vi "Filter And Analyze.vi"(9 "X Resolution":i32, 10 "Y Resolution":i32, 11 "Refnum in":T1) -> (0 "Number of Particles":i32, 1 "Particle Reports (Pixels)":T3(array[cluster]) {"Orientation" format="%.2f"; "Dimensions"."Height" format="%.2f"; "Dimensions"."Width" format="%.2f"; "Center of Mass"."Y" format="%.2f"; "Center of Mass"."X" format="%.2f"; "Bounding Rect"."Bottom" format="%.2f"; "Bounding Rect"."Right" format="%.2f"; "Bounding Rect"."Top" format="%.2f"; "Bounding Rect"."Left" format="%.2f"; "Number of Holes" format="%.2f"; "Area" format="%.2f"}, 3 "Filtered Array":T2(array[cluster]))   [LabVIEW 2012]
uses:
  <vilib>/vision/Image Controls.llb/IMAQ Image.ctl
  <vilib>/vision/NI_Vision_Development_Module.lvlib
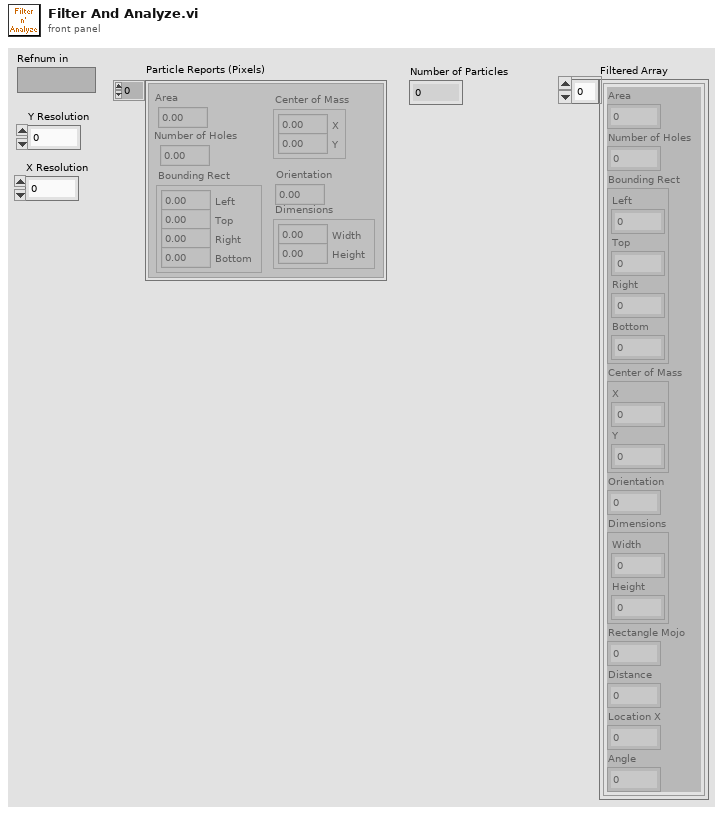
[diagram p1: front panel]
types:
  T1 = typedef "IMAQ Image.ctl" = refnum<image>
  T2 = cluster{"Area":dbl, "Number of Holes":dbl, "Bounding Rect":cluster{"Left":dbl, "Top":dbl, "Right":dbl, "Bottom":dbl}, "Center of Mass":cluster{"X":dbl, "Y":dbl}, "Orientation":dbl, "Dimensions":cluster{"Width":dbl, "Height":dbl}, "Rectangle Mojo":dbl, "Distance":dbl, "Location X":dbl, "Angle":dbl}[]
  T3 = cluster{"Area":dbl, "Number of Holes":dbl, "Bounding Rect":cluster{"Left":dbl, "Top":dbl, "Right":dbl, "Bottom":dbl}, "Center of Mass":cluster{"X":dbl, "Y":dbl}, "Orientation":dbl, "Dimensions":cluster{"Width":dbl, "Height":dbl}}[]
  T4 = cluster{"Area":dbl, "Number of Holes":dbl, "Bounding Rect":cluster{"Left":dbl, "Top":dbl, "Right":dbl, "Bottom":dbl}, "Center of Mass":cluster{"X":dbl, "Y":dbl}, "Orientation":dbl, "Dimensions":cluster{"Width":dbl, "Height":dbl}, "Rectangle Mojo":dbl, "Distance":dbl, "Location X":dbl, "Angle":dbl}
  T5 = typedef "Particle Parameters" = i32
  T6 = cluster{"Measurement Parameter":T5, "Range Lower Value":dbl, "Range Upper Value":dbl, "Range":bool, "Measurement Type":bool}[]
  T7 = typedef "Image Type" = u32
  T8 = cluster{"Left":dbl, "Top":dbl, "Right":dbl, "Bottom":dbl}
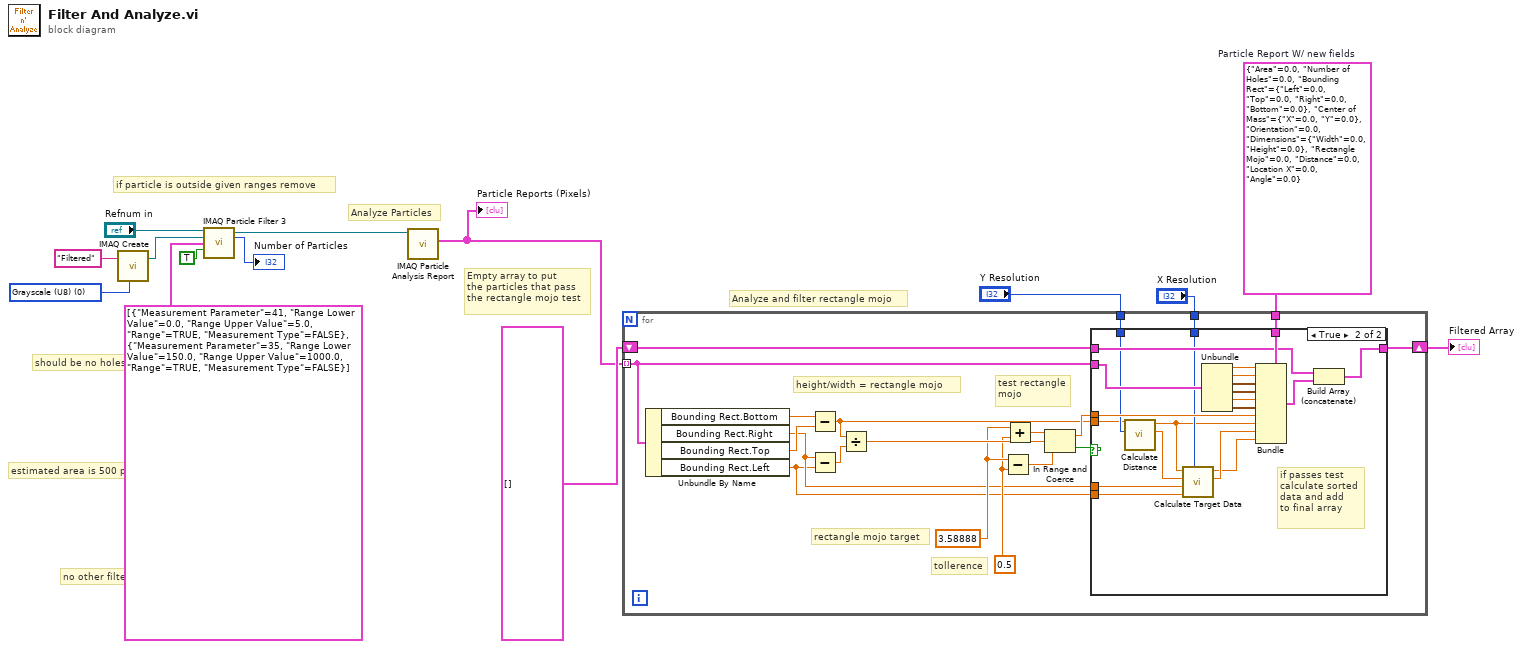
[diagram p0: block diagram]
diagram:
  w10 = T4 {"Area"=0.0, "Number of Holes"=0.0, "Bounding Rect"={"Left"=0.0, "Top"=0.0, "Right"=0.0, "Bottom"=0.0}, "Center of Mass"={"X"=0.0, "Y"=0.0}, "Orientation"=0.0, "Dimensions"={"Width"=0.0, "Height"=0.0}, "Rectangle Mojo"=0.0, "Distance"=0.0, "Location X"=0.0, "Angle"=0.0}  # Particle Report W/ new fields
  w3 = T7 0 items=["Grayscale (U8)", "Grayscale (I16)", "Grayscale (SGL)", "Complex (CSG)", "RGB (U32)", "HSL (U32)", "RGB (U64)", "Grayscale (U16)"] ("Image Type")
  # "Empty array to put\nthe particles that pass\nthe rectangle mojo test"
  # "Analyze and filter rectangle mojo"
  # "Analyze Particles"
  # "no other filter"
  # "should be no holes"
  # "if particle is outside given ranges remove"
  # "estimated area is 500 px"
  n1 = call "IMAQ Create"("Image Name"="Filtered", "Image Type"=w3) -> ("New Image"=w5:T1)  [unwired: 3 in, 1 out]
  n2 = call "IMAQ Particle Filter 3"("Image Src"="Refnum in", "Image Dst"=w5, "Selection Values"=T6 [{"Measurement Parameter"=41, "Range Lower Value"=0.0, "Range Upper Value"=5.0, "Range"=TRUE, "Measurement Type"=FALSE}, {"Measurement Parameter"=35, "Range Lower Value"=150.0, "Range Upper Value"=1000.0, "Range"=TRUE, "Measurement Type"=FALSE}], "Keep/Remove Particles (F)"=TRUE) -> ("Image Dst Out"=w2:T1, "Number of Particles"=→"Number of Particles":i32)  [unwired: 9 in, 1 out]
  n3 = call "IMAQ Particle Analysis Report"("Image"=w2) -> ("Particle Reports (Pixels)"=w9:T3)  [unwired: 5 in, 5 out]
  "Particle Reports (Pixels)" <- w9
  n4 = for {
    tunnel: w9 -> [w27] mode=indexing
    tunnel: w10 -> [w26]
    tunnel: "Y Resolution" -> [w24]
    shift-right: [w23] -> w14
    shift-left: T2 [] -> [w22]
    tunnel: "X Resolution" -> [w21]
    w29 = 0.5 ("upper limit")
    w30 = 3.58888 ("upper limit")
    # "test rectangle\nmojo"
    # "tollerence"
    # "rectangle mojo target"
    # "height/width = rectangle mojo"
    n5 = Unbundle By Name(w27) -> ("Bounding Rect.Bottom"=w20:dbl, "Bounding Rect.Right"=w16:dbl, "Bounding Rect.Top"=w19:dbl, "Bounding Rect.Left"=w15:dbl)
    n6 = Subtract(x=w20, y=w19) -> (x-y=w17:dbl)
    n7 = Subtract(x=w16, y=w15) -> (x-y=w18:dbl)
    n8 = Divide(x=w17, y=w18) -> (x/y=w33:dbl)
    n9 = Subtract(x=w30, y=w29) -> (x-y=w31:dbl)
    n10 = Add(x=w30, y=w29) -> (x+y=w32:dbl)
    n11 = In Range and Coerce(upper limit=w32, x=w33, lower limit=w31) -> (coerced(x)=w25:dbl, In Range?=w28:bool)
    n12 = case shown="True" w28 {
      tunnel: w27 -> [_ w53]
      tunnel: [w34 w55] -> w23
      tunnel: w22 -> [w34 w44]
      tunnel: w26 -> [_ w54]
      tunnel: w25 -> [_ w46]
      tunnel: w24 -> [_ w43]
      tunnel: w21 -> [_ w42]
      tunnel: w17 -> [_ w37]
      tunnel: w16 -> [_ w36]
      tunnel: w15 -> [_ w35]
      frame False {
        # "if fails test don't add\nto final array"
      }
      frame True {
        # "if passes test\ncalculate sorted\ndata and add\nto final array"
        n13 = call "Calculate Distance.vi"("Y Resolution"=w43, "Target Height (px)"=w37) -> ("real size to pixle ration (in/px)"=w40:dbl, "Distance (in)"=w41:dbl)  [unwired: 8 in]
        n14 = call "Calculate Target Data.vi"("X resolution"=w42, "Rect Left"=w35, "Rect Right"=w36, "Real size to pixle ratio (in/px)"=w40, "Distance to Target (in)"=w41) -> ("X Location (in)"=w39:dbl, "Angle"=w38:dbl)  [unwired: 5 in]
        n15 = Unbundle(w53) -> ("Area"=w52:dbl, "Number of Holes"=w51:dbl, "Bounding Rect"=w50:T8, "Center of Mass"=w49:cluster{"X":dbl, "Y":dbl}, "Orientation"=w48:dbl, "Dimensions"=w47:cluster{"Width":dbl, "Height":dbl})
        n16 = Bundle(cluster=w54, "Area"=w52, "Number of Holes"=w51, "Bounding Rect"=w50, "Center of Mass"=w49, "Orientation"=w48, "Dimensions"=w47, "Rectangle Mojo"=w46, "Distance"=w41, "Location X"=w39, "Angle"=w38) -> (w45:T4)
        n17 = Build Array (concatenate)(w44, w45) -> (w55:T2)
      }
    }
  }
  "Filtered Array" <- w14
